vi "4) Programa Graficación.vi"() -> ()   [LabVIEW 2014]
panel:
  in  "Estados de los canales":T1
  out "error out":errorcluster
  out "VISA resource name out":refnum<visa-resource-name>
  in  "VISA resource name":refnum<visa-resource-name>
  out "Gráfica":waveform(dbl)[](graph)
  in  "error in (no error)":errorcluster
  in  "Punto final de la onda":i32=2500 min=0 max=2500 step=1
  in  "Punto inicial de la onda":i32 min=0 max=2500 step=1
  in  "Mayor Precisión":bool
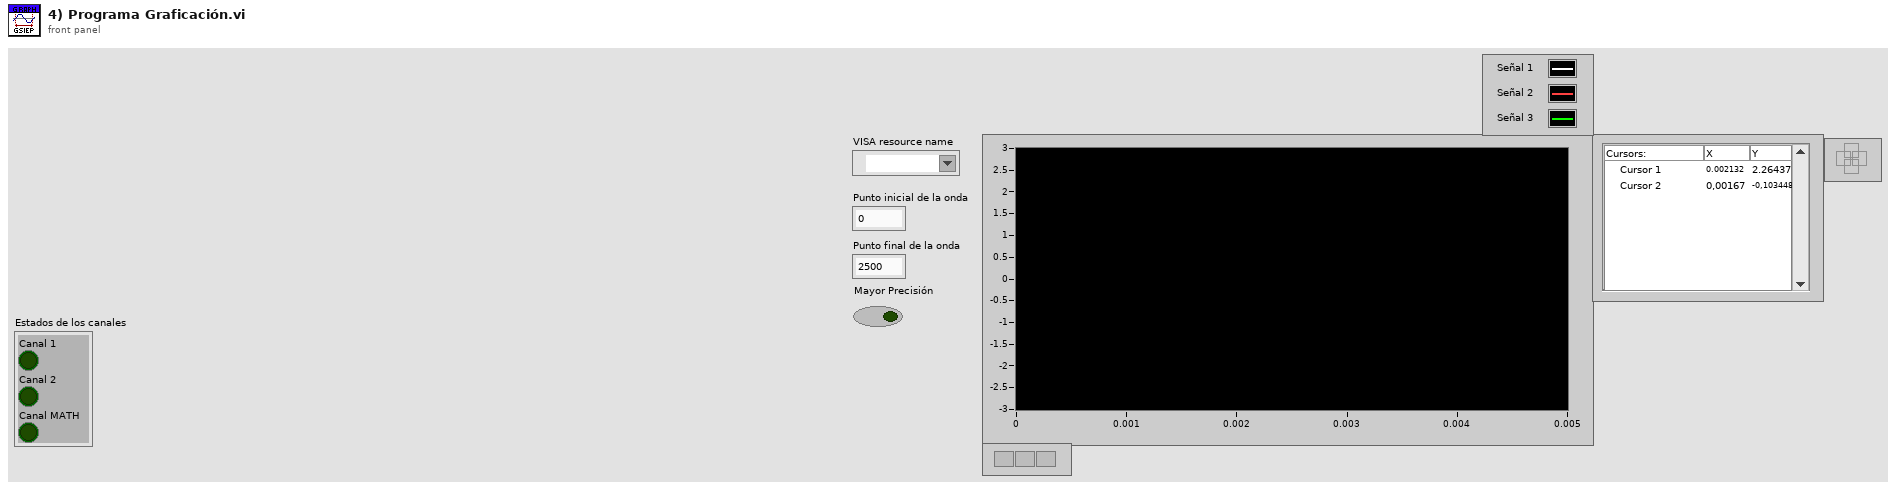
[diagram p1: front panel]
types:
  T1 = cluster{"Canal 1":bool, "Canal 2":bool, "Canal MATH":bool}
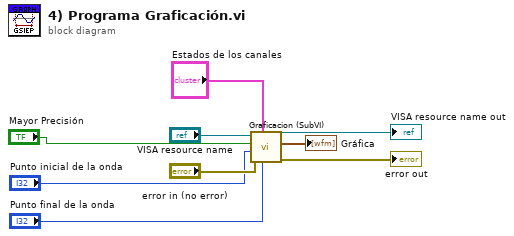
[diagram p0: block diagram]
diagram:
  n1 = call "Graficacion (SubVI).vi"("Punto final de la onda"="Punto final de la onda", "Estados de los canales"="Estados de los canales", "error in (no error)"="error in (no error)", "Punto inicial de la onda"="Punto inicial de la onda", "Mayor Precisión"="Mayor Precisión", "VISA Refnum in"="VISA resource name") -> ("error out"=→"error out":errorcluster, "Gráfica"=→"Gráfica":waveform(dbl)[], "VISA Refnum out"=→"VISA resource name out":refnum<visa-resource-name>)  [unwired: 3 in]
